vi "LIDAR data processing.vi"(9 "LIDAR raw data":u8) -> (1 "driveable path lengths":u16[](array[numeric]), 2 "angle":u8, 3 "last measured value":u16)   [LabVIEW 2010]
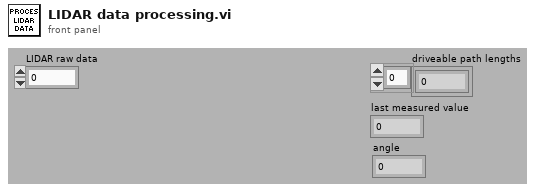
[diagram p1: front panel]
types:
  T1 = enum16{"confirm check sum", "check status byte", "read measured values", "confirm measurement", "confirm command", "read message length", "read address", "wait for \"02\""}
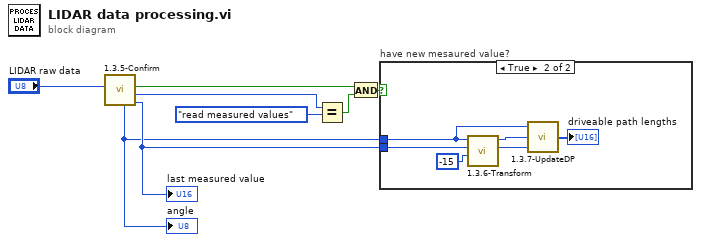
[diagram p0: block diagram]
diagram:
  n1 = call "1.3.5-Confirm.vi"("LIDAR raw data"="LIDAR raw data") -> ("last measured value"=w3:u16, "parser state"=w5:T1, "new value?"=w6:bool, "angle"=w2:u8)  [unwired: 7 in]
  "last measured value" <- w3
  "angle" <- w2
  n2 = Equal?(x=w5, y=T1."read measured values" ("parser state")) -> (x = y?=w8:bool)
  n3 = And(x=w6, y=w8) -> (x .and. y?=w4:bool)
  n4 = case "have new mesaured value?" shown="True" w4 {
    tunnel: w3 -> [_ w14]
    tunnel: w2 -> [_ w10]
    frame False {
    }
    frame True {
      n5 = call "1.3.6-Transform.vi"("Lidar Vertical Position"=i8 -15, "Lidar Distance"=w14, "Lidar Scan Angle"=w10) -> ("Robot Y"=w11:i16, "Lidar X = Robot X"=w12:i16)  [unwired: 3 in, 4 out]
      n6 = call "1.3.7-UpdateDP.vi"("Robot Y"=w11, "Robot X"=w12, "Lidar Angle"=w10) -> ("driveable path lengths"=→"driveable path lengths":u16[])  [unwired: 2 in]
    }
  }
